vi "Test_Rename_And_Set_Value.vi"   [LabVIEW 2025]
uses:
  8cebb4ce-4f0f-4319-9f7e-82e401bee674.vi
  0e244da9-745b-4f2d-a97c-0de3ccfbb071.vi
  57ba1f44-eecb-4af5-975d-0cda700306c1.vi
  Scripting Server.lvlib
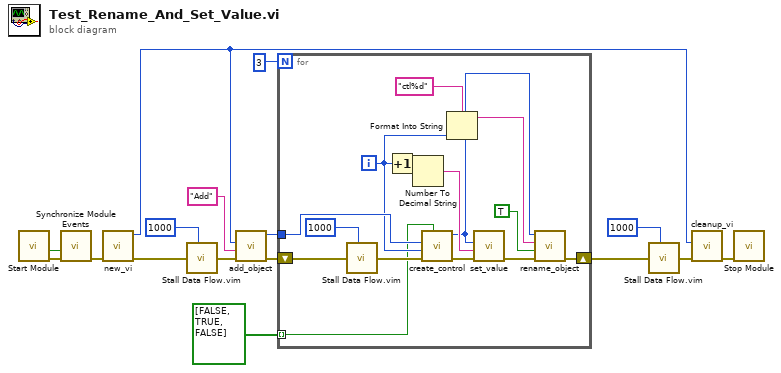
[diagram p0: block diagram]
diagram:
  n1 = call "Start Module.vi"() -> ("error out"=w15:errorcluster, "Wait for Event Sync?"=w16:bool)  [unwired: 7 in, 3 out]
  n2 = call "Synchronize Module Events.vi"("error in"=w15, "Wait for Event Sync?"=w16) -> ("error out"=w14:errorcluster)  [unwired: 9 in]
  n3 = call "new_vi.vi"("error in"=w14) -> ("error out"=w13:errorcluster, "vi_id"=w5:i32)  [unwired: 7 in, 2 out]
  n4 = call "Stall Data Flow.vim"("value in"=w13, "milliseconds to wait"=u32 1000) -> ("value out"=w12:errorcluster)  [unwired: 1 out]
  n5 = call "add_object.vi"("error in"=w12, "object_name"="Add", "vi_reference"=w5) -> ("error out"=w10:errorcluster, "object_id"=w9:i32)  [unwired: 5 in, 2 out]
  n6 = for {
    N: 3 -> [_]
    tunnel: w9 -> [w30]
    shift-right: [w24] -> w6
    shift-left: w10 -> [w31]
    tunnel: bool[] [FALSE, TRUE, FALSE] ("constant") -> [w18] mode=indexing
    i -> [w21]
    n7 = call "Stall Data Flow.vim"("value in"=w31, "milliseconds to wait"=u32 1000) -> ("value out"=w29:errorcluster)  [unwired: 1 out]
    n8 = Increment(x=w21) -> (x+1=w17:i32)
    n9 = Number To Decimal String(number=w17) -> (decimal integer string=w25:string)  [unwired: 1 in]
    n10 = call "create_control.vi"("constant"=w18, "error in"=w29, "terminal_index"=w21, "object_id"=w30) -> ("error out"=w27:errorcluster, "created_object_id"=w23:i32)  [unwired: 5 in, 1 out]
    n11 = Format Into String(format string="ctl%d", w21) -> (resulting string=w20:string)  [unwired: 2 in, 1 out]
    n12 = call "set_value.vi"("error in"=w27, "value"=w25, "object_id"=w23) -> ("error out"=w26:errorcluster)  [unwired: 7 in, 1 out]
    n13 = call "rename_object.vi"("error in"=w26, "label_visible"=TRUE, "new_label_name"=w20, "object_id"=w23) -> ("error out"=w24:errorcluster)  [unwired: 6 in, 1 out]
  }
  n14 = call "Stall Data Flow.vim"("value in"=w6, "milliseconds to wait"=u32 1000) -> ("value out"=w4:errorcluster)  [unwired: 1 out]
  n15 = call "cleanup_vi.vi"("error in"=w4, "vi_reference"=w5) -> ("error out"=w2:errorcluster)  [unwired: 7 in, 2 out]
  n16 = call "Stop Module.vi"("error in"=w2) -> ()  [unwired: 10 in, 1 out]
